vi "Process-Ethernet-Frames.vi"(10 "Source Machine\nSettings":T1={"MAC Address"=[0, 1, 2, 3, 4, 5], "IP Address"=[10, 0, 1, 101]} {"MAC Address" format="%.0x"}, 11 "Raw Data\nStream":u64[](array[numeric])=[68719476735, 68719411202, 67802302532, 64559120385, 64558728708, 64424574978, 67802302532, 64592281956, 64424509440, 64424512000, 64447905792, 64424509440, 64424509440, 64424509440, 64424509440, 66519609314, 281539401220098, 68719476735, 68719411202, 67802302532, 64559120385, 64558728708, 64424574978, 67802302532, 64592281956, 64424509440, 64424512000, 64447905792, 64424509440, 64424509440, 64424509440, 64424509440, 66519609314, 281539401220098, 68719476735, 68719411202, 67802302532, 64559120385, 64558728708, 64424574978, 67802302532, 64592281956, 64424509440, 64424512000, 64447905792, 64424509440, 64424509440, 64424509440, 64424509440, 66519609314, 281539401220098] format="%.0x") -> (1 "UDP Payload":u8[](array[numeric]) format="%.0x", 2 "Messages":string[](array[string]), 3 "Frames to send":u8[][](array[numeric]) format="%.0x")   [LabVIEW 2017]
uses:
  Source.Machine.Settings.ctl
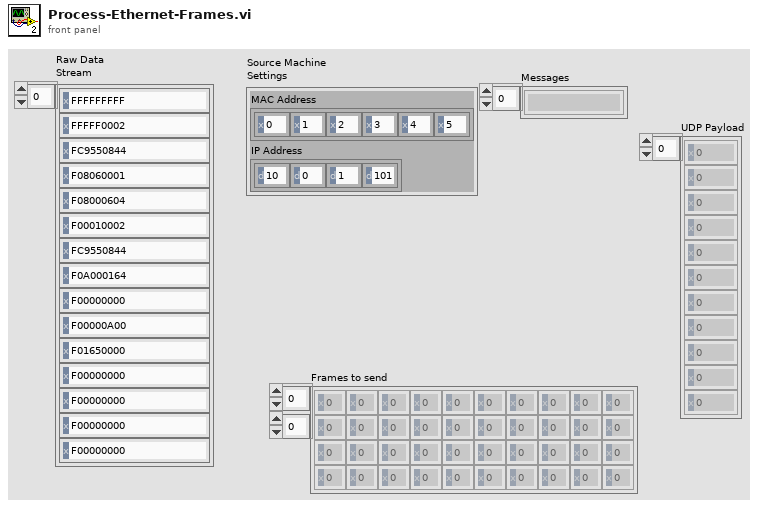
[diagram p1: front panel]
types:
  T1 = typedef "Source.Machine.Settings.ctl" = cluster{"MAC Address":u8[], "IP Address":u8[]}
  T2 = cluster{"Version":u8, "Header Length":u8, "Total Length":u16, "More Fragments":bool, "Don't Fragment":bool, "Fragment Offset":u16, "TTL":u8, "Header Checksum":u16, "Identification":u16, "Protocol":u8, "Source IP":u8[], "Destination IP":u8[]}
  T3 = cluster{"Type of Message":u8, "Code":u8, "Checksum":u16, "Quench":u32}
  T4 = typedef "Source.Machine.Settings" = cluster{"MAC Address":u8[], "IP Address":u8[]}
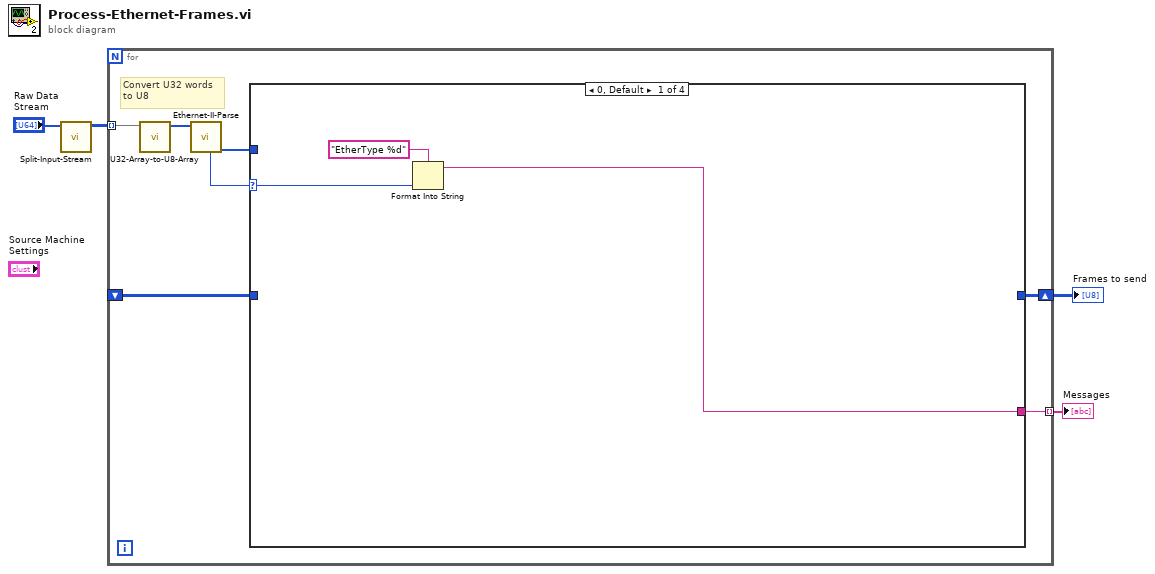
[diagram p0: block diagram]
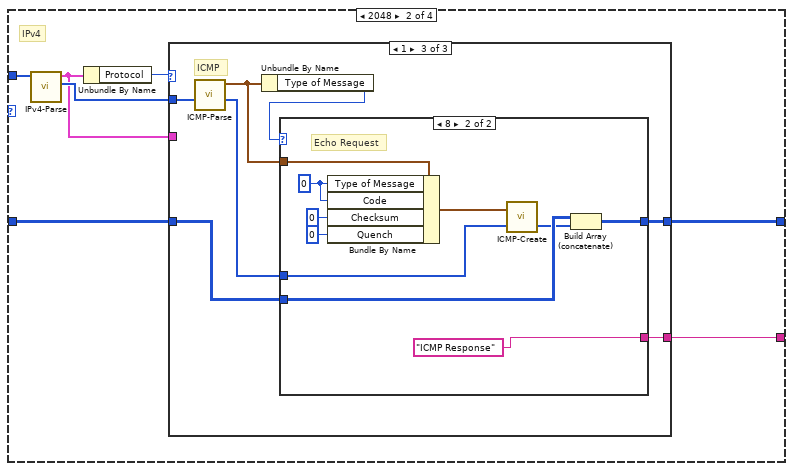
[diagram p2: hidden frame]
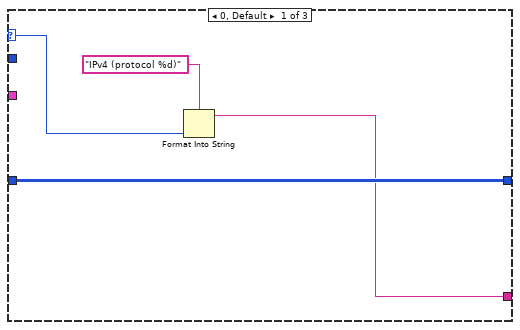
[diagram p3: hidden frame]
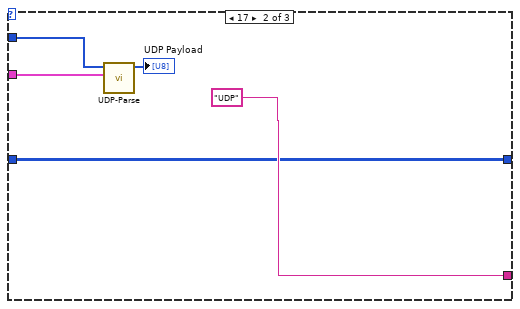
[diagram p4: hidden frame]
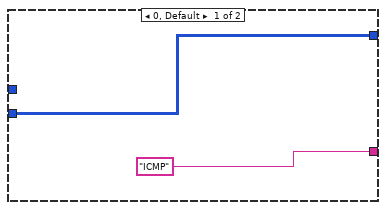
[diagram p5: hidden frame]
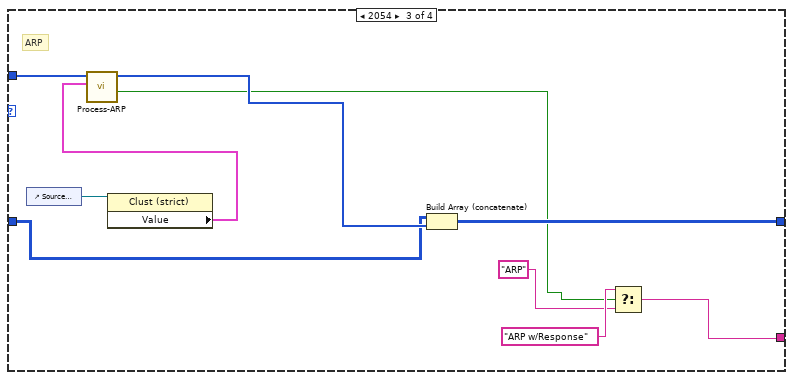
[diagram p6: hidden frame]
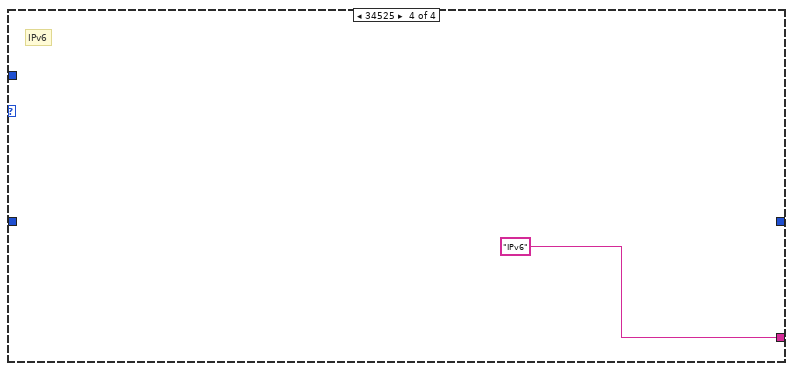
[diagram p7: hidden frame]
diagram:
  n1 = call "Split-Input-Stream.vi"("Raw Data\nStream"="Raw Data\nStream") -> ("Array"=w3:u32[][])  [unwired: 10 in]
  n2 = for {
    tunnel: w3 -> [w11] mode=indexing
    shift-right: [w7] -> w2
    shift-left: _ -> [w6]
    tunnel: [w5] -> w1 mode=indexing
    # "Convert U32 words\nto U8"
    n3 = call "U32-Array-to-U8-Array.vi"("U32 [] in"=w11) -> ("U8 [] out"=w10:u8[])  [unwired: 10 in]
    n4 = call "Ethernet-II-Parse.vi"("Input Frame"=w10) -> ("Payload"=w8:u8[], "EtherType"=w9:u16)  [unwired: 6 in, 3 out]
    n5 = case shown="0, Default" w9 {
      selector: w9 -> [w13 _ _ _]
      tunnel: w8 -> [_ w21 w59 _]
      tunnel: [_ w18 w56 _] -> w7
      tunnel: w6 -> [_ w17 w55 _]
      tunnel: [w12 w16 w50 "IPv6"] -> w5
      frame 0, Default {
        n6 = Format Into String(format string="EtherType %d", w13) -> (resulting string=w12:string)  [unwired: 2 in, 1 out]
      }
      frame 2048 {
        # "IPv4"
        n7 = call "IPv4-Parse.vi"("IPv4 Packet (in)"=w21) -> ("IPv4 Payload"=w19:u8[], "Header"=w15:T2)  [unwired: 8 in, 1 out]
        n8 = Unbundle By Name(w15) -> ("Protocol"=w20:u8)
        n9 = case shown="1" w20 {
          selector: w20 -> [w23 _ _]
          tunnel: w19 -> [_ w30 w37]
          tunnel: [w25 w26 w33] -> w18
          tunnel: w17 -> [w25 w26 w32]
          tunnel: [w22 "UDP" w31] -> w16
          tunnel: w15 -> [_ w29 _]
          frame 0, Default {
            n10 = Format Into String(format string="IPv4 (protocol %d)", w23) -> (resulting string=w22:string)  [unwired: 2 in, 1 out]
          }
          frame 17 {
            n11 = call "UDP-Parse.vi"("IPv4 Header"=w29, "UDP Packet"=w30) -> ("UDP Payload"=→"UDP Payload":u8[])  [unwired: 9 in]
          }
          frame 1 {
            # "ICMP"
            n12 = call "ICMP-Parse.vi"("IPv4 Payload"=w37) -> ("Data"=w34:u8[], "Header"=w35:T3)  [unwired: 8 in, 1 out]
            n13 = Unbundle By Name(w35) -> ("Type of Message"=w36:u8)
            n14 = case shown="8" w36 {
              tunnel: w35 -> [_ w49]
              tunnel: w34 -> [_ w44]
              tunnel: [w39 w43] -> w33
              tunnel: w32 -> [w39 w42]
              tunnel: ["ICMP" "ICMP Response"] -> w31
              frame 0, Default {
              }
              frame 8 {
                w48 = u8 0 ("Type of Message")
                # "Echo Request"
                n15 = Bundle By Name(cluster=w49, "Type of Message"=w48, "Code"=w48, "Checksum"=u16 0, "Quench"=u32 0) -> (w45:T3)
                n16 = call "ICMP-Create.vi"("Payload"=w44, "Header"=w45) -> ("ICMP Message"=w41:u8[])  [unwired: 1 in]
                n17 = Build Array (concatenate)(w42, w41) -> (w43:u8[][])
              }
            }
          }
        }
      }
      frame 2054 {
        # "ARP"
        n18 = control-ref of="Source Machine\nSettings"() -> (w58:refnum<vi>)
        n19 = property class="Clust (strict)"(reference=w58) -> ("Value"=w54:T4)  [unwired: 1 in, 2 out]
        n20 = call "Process-ARP.vi"("Source Machine\nSettings"=w54, "Frame (in)"=w59) -> ("Response\nNeeded?"=w52:bool, "ARP Response"=w57:u8[])  [unwired: 8 in]
        n21 = Build Array (concatenate)(w55, w57) -> (w56:u8[][])
        n22 = Select(t="ARP w/Response", s=w52, f="ARP") -> (s? t:f=w50:string)
      }
      frame 34525 {
        # "IPv6"
      }
    }
  }
  "Frames to send" <- w2
  "Messages" <- w1
